vi "子界面-查看某框和报告生成.vi"(2 "测试人":string, 4 "标注图":T1(plugin-control), 5 "部位":string, 6 "产品序号":string, 7 "反射图":T1(plugin-control), 8 "框组":T5(array[cluster]), 9 "框号":dbl format="%#_13g") -> ()   [LabVIEW 2018]
uses:
  <vilib>/addons/database/Connection.llb/DB Tools Open Connec (String).vi
  <vilib>/vision/NI_Vision_Development_Module.lvlib
  <vilib>/addons/database/NI_Database_API.lvlib
panel:
  out "反射图ROI对应区域灰度表":u32[](graph)
  out "?":T1(plugin-control)
  out "Threshold Image":T1(plugin-control)
  out "分层类检测结果":string[][](table)
  out "Threshold Image":T1(plugin-control)
  out "Threshold Image":T1(plugin-control)
  out "反射图ROI的最大灰度值":sgl
  in  "反射法图像-面积阈值设置":T3(array[cluster]) {"Measurement Parameter" items=["Area"]; "下限" min=0 step=1; "上限" min=0 step=1}
  in  "灰度阈值设置":cluster{"下限":dbl, "下限":dbl}(slide)={"下限"=0.0, "下限"=65.10638427734375} scale=0.0..255.0
  in  "保存结果":bool
  in  "Color":u32[](array[colorbox])=[3381759, 16776770, 16777225, 6618880]
  in  "Overlay Type":u16[](array[ring])=[2, 1, 3, 0] items=["Rectangle", "Numbers", "Points", "Lines"]
  in  "Tab Control":T4(tab)
  out "穿透ROI":T1(plugin-control)
  out "Threshold Image":T1(plugin-control)
  out "?":T1(plugin-control)
  out "?":T1(plugin-control)
  out "Threshold Image":T1(plugin-control)
  out "Threshold Image":T1(plugin-control)
  out "弥散测量结果":dbl[][](array[numeric]) format="%.2f"
  in  "分隔符（'\\'代码显示）":string="\t"
  in  "格式字符串":string="%f"
  out "弥散类检测结果":string[][](table)
  out "?":string
  out "面积 (pixels)":i32
  out "写入数据库路径":path
  out "Z值 2":dbl[](array[numeric])
  out "Z值":dbl[](array[numeric])
  out "tables":string[](array[string])
  in  "写入数据库":bool
  out "ROI位置Y":i32
  out "ROI位置X":i32
  out "报告生成路径":path
  in  "格式字符串 2":string="%f"
  in  "分隔符（'\\'代码显示）":string="\t"
  out "分层测量结果":dbl[][](array[numeric]) format="%.2f"
  out "缺陷分类的临界值":sgl format="%#.3f"
  in  "返回 2":bool
  in  "报告生成":bool
  # "所选区域信息"
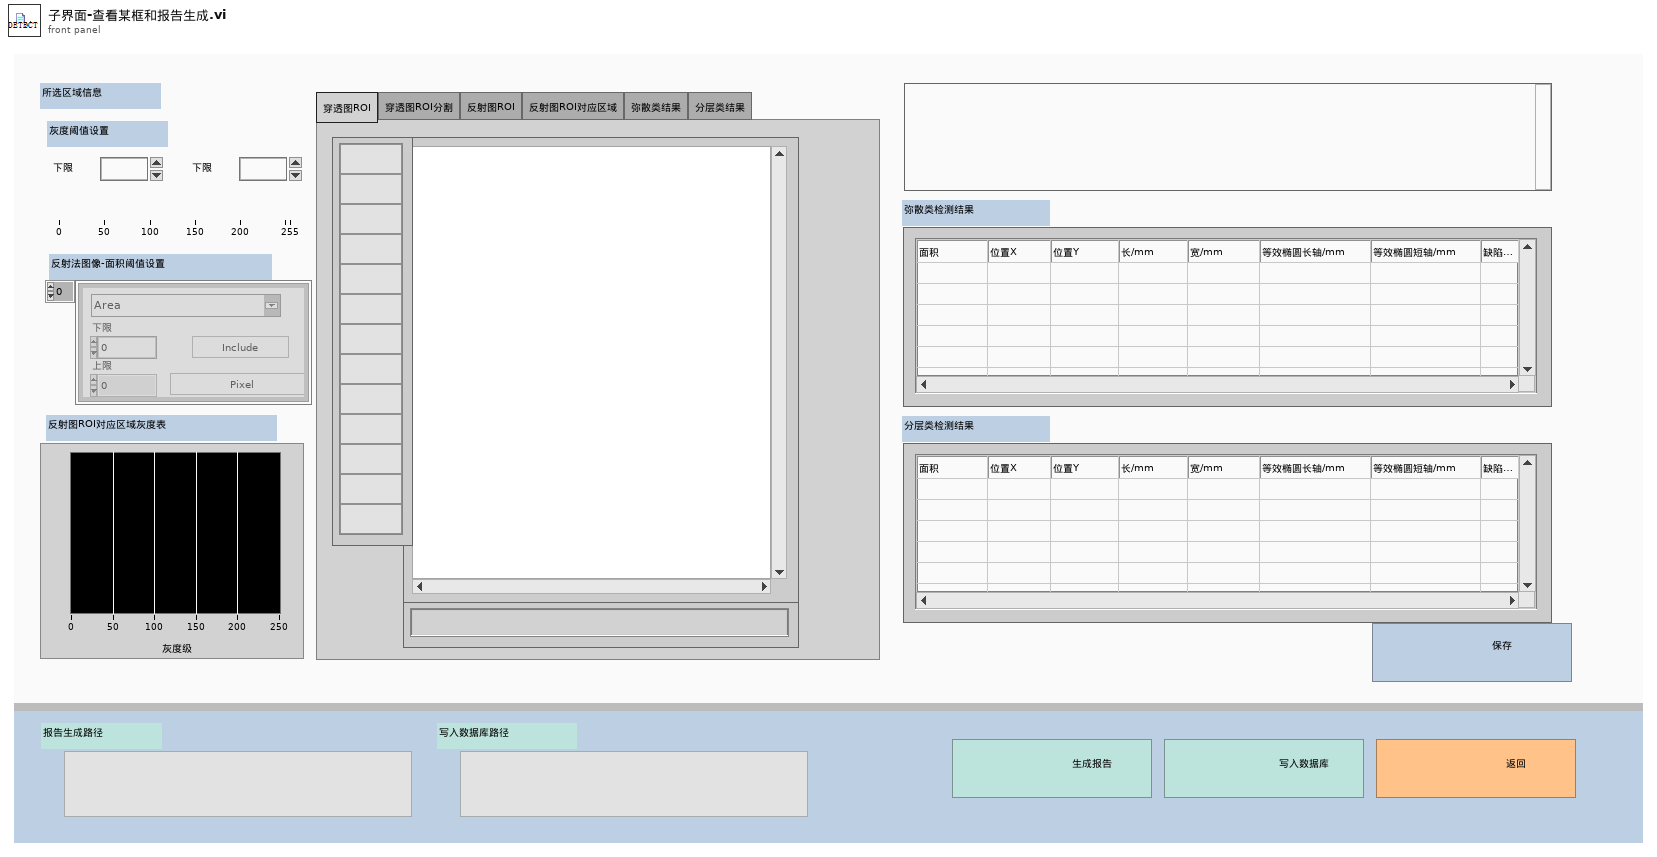
[diagram p1: front panel]
types:
  T1 = typedef "IMAQ Image.ctl" = refnum<image>
  T2 = typedef "Particle Parameters" = i32
  T3 = cluster{"Measurement Parameter":T2, "下限":i32, "上限":i32, "Range":bool, "Measurement Type":bool}[]
  T4 = enum32{"穿透图ROI", "穿透图ROI分割", "反射图ROI", "反射图ROI对应区域", "弥散类结果", "分层类结果"}
  T5 = cluster{"Global Rectangle":i32[], "Contours":cluster{"Contour Type":u32, "ROI Type":u32, "Points":i32[]}[]}[]
  T6 = typedef "Image Type" = u32
  T7 = cluster{"Global Rectangle":i32[], "Contours":cluster{"Contour Type":u32, "ROI Type":u32, "Points":i32[]}[]}
  T8 = cluster{"Pixel Measurements":T2[], "Overlay Type":u16[], "Color":u32[], "反射法图像-面积阈值设置":cluster{"Measurement Parameter":T2, "下限":i32, "上限":i32, "Range":bool, "Measurement Type":bool}[], "灰度阈值设置":cluster{"下限":dbl, "下限":dbl}}
  T9 = cluster{"histogram":u32[], "Minimal Value":sgl, "Maximal Value":sgl, "Starting Value":sgl, "Interval Width":sgl, "Mean Value":sgl, "Standard  Variation":sgl, "Area (pixels)":i32}
  T10 = cluster{"Desired Font (Application)":enum16{"User-specified Font", "Application Font", "System Font", "Dialog Font"}, "[User-specified Font]":cluster{"Font Name":string, "Size":i16, "Strikeout?":bool, "Italic?":bool, "Underline?":bool, "Outline?":bool, "Shadow?":bool, "Bold?":bool, "Rotation Angle":dbl}, "Horizontal Alignment":i16, "Vertical Alignment":i16}
  T11 = typedef "NI_Database_API.lvlib/Conn ObjectReference.ctl" = refnum<k1>
  T12 = cluster{"框号":dbl, "Numeric":dbl, dbl, dbl, "Numeric":dbl, "Numeric":dbl, "Numeric":dbl, "Numeric":dbl, "数值":dbl, string}
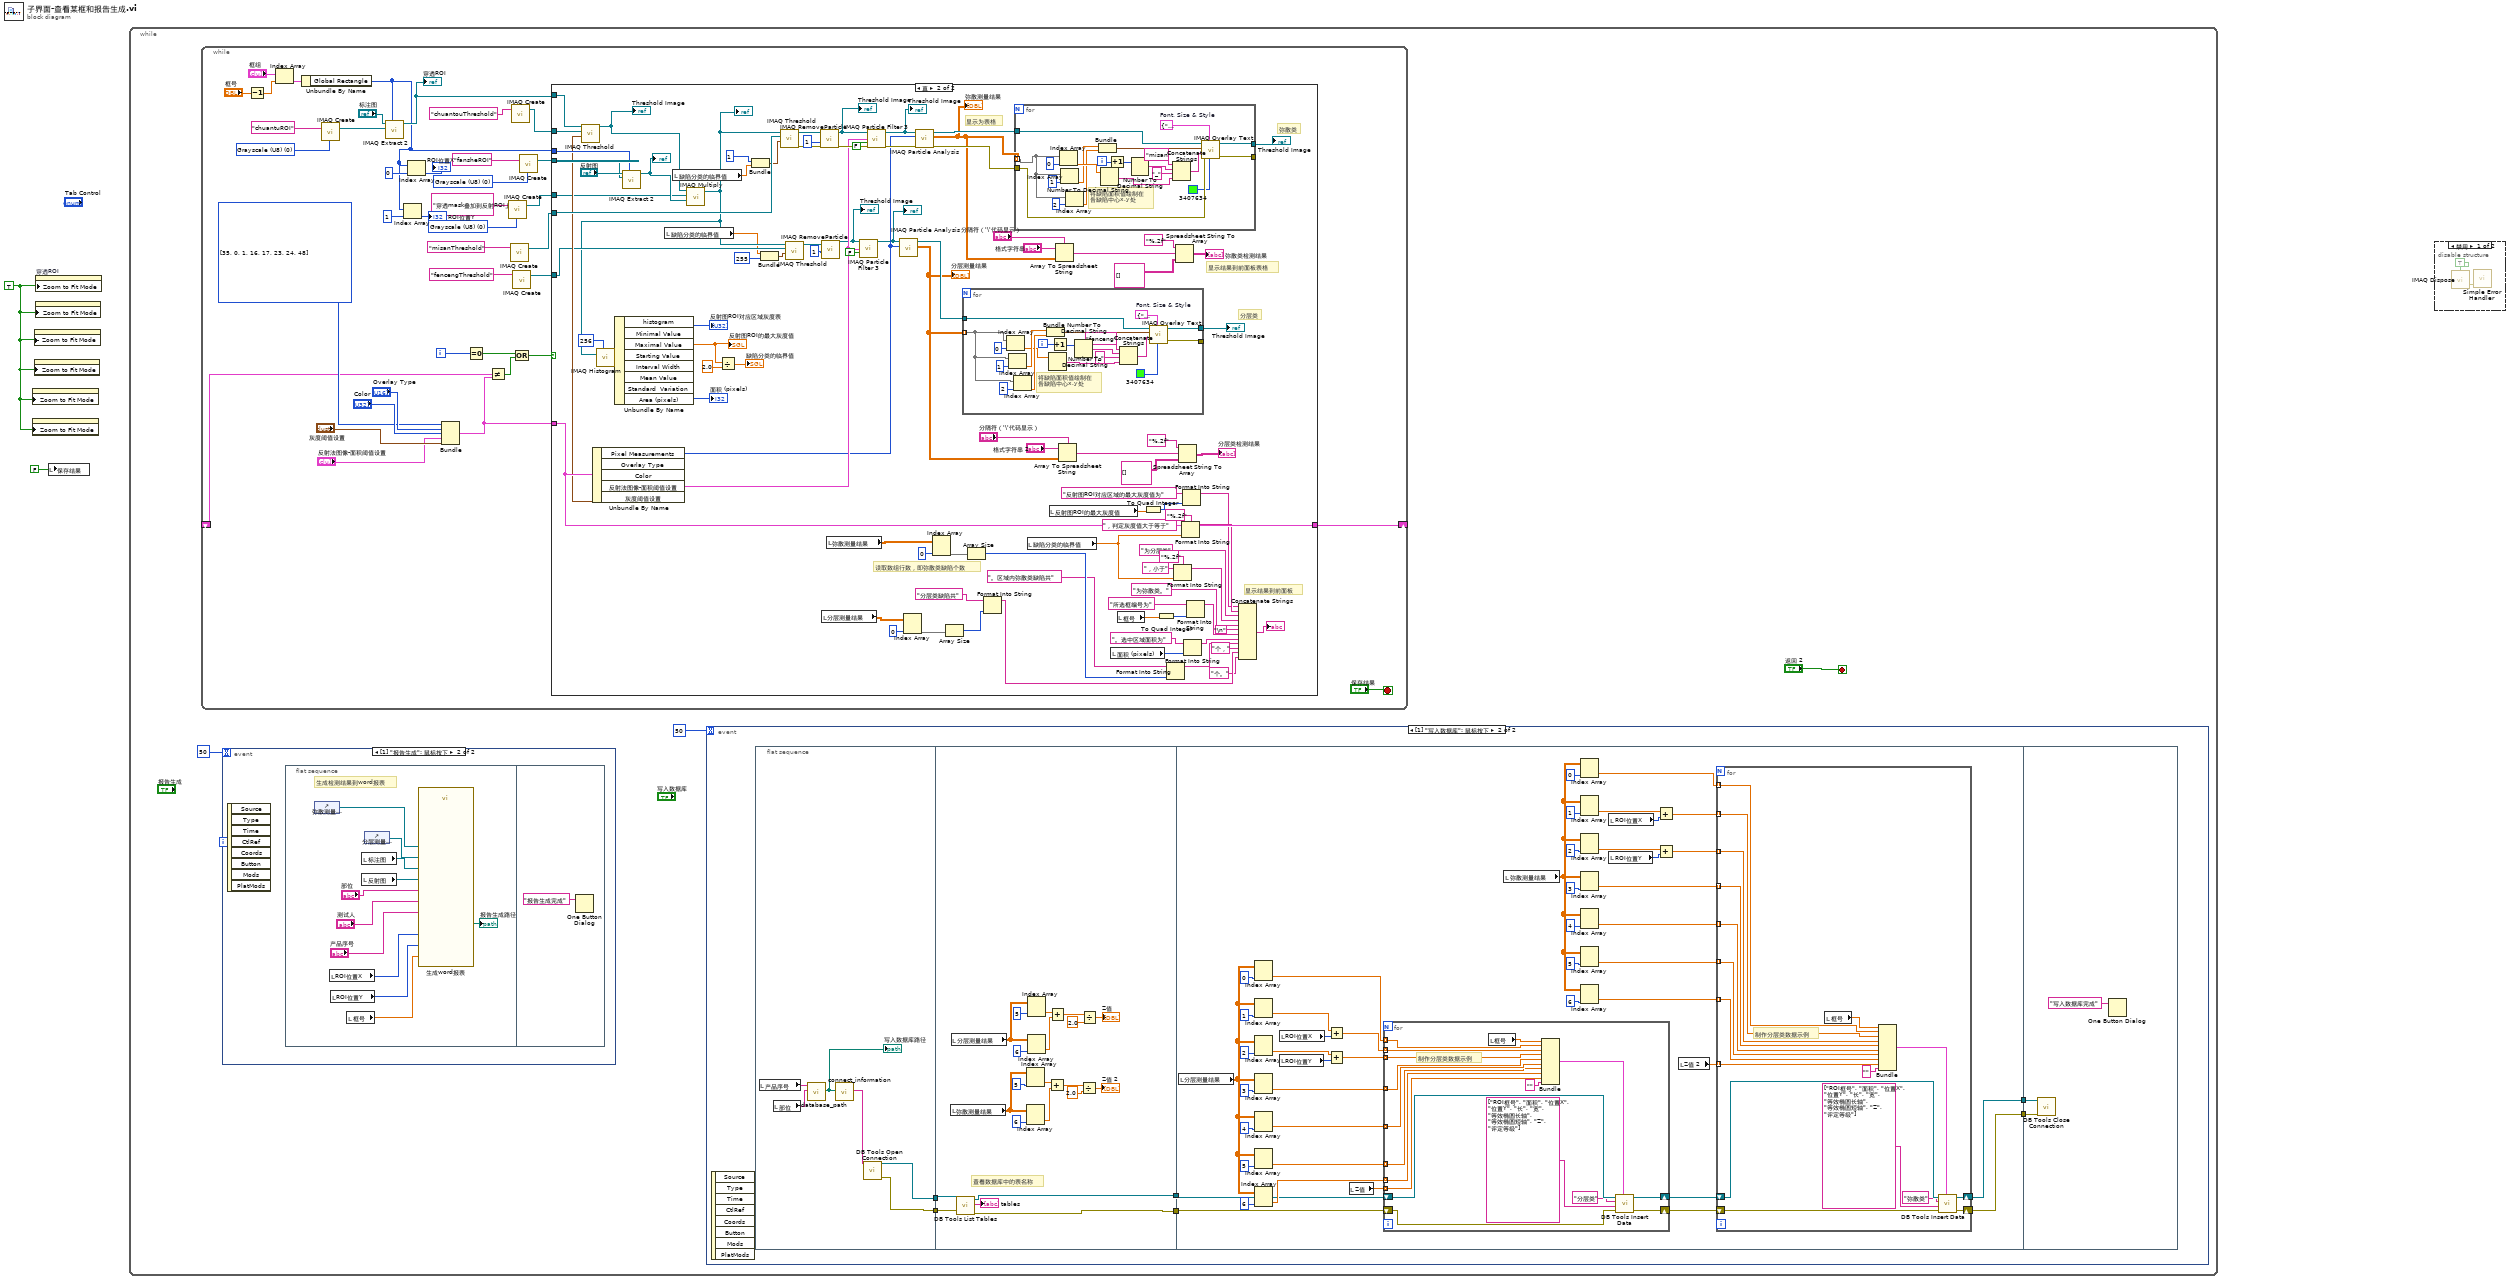
[diagram p0: block diagram]
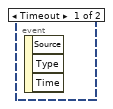
[diagram p3: hidden frame]
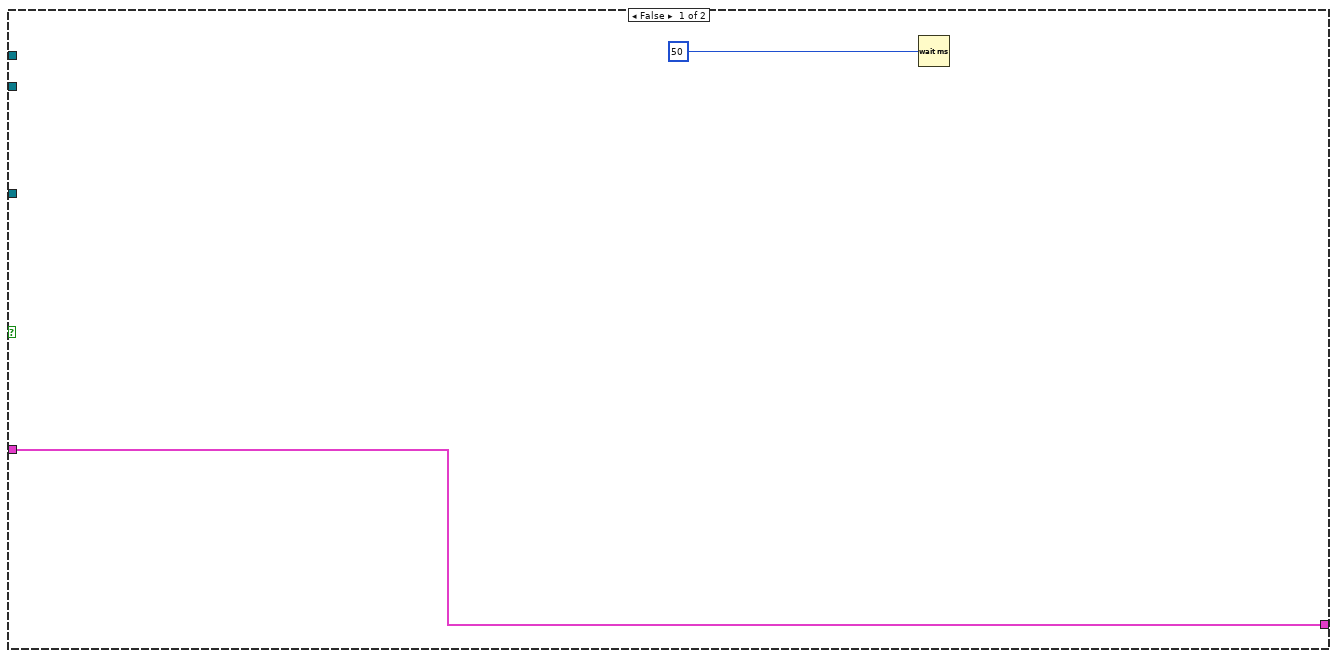
[diagram p4: hidden frame]
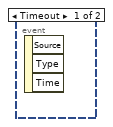
[diagram p5: hidden frame]
diagram:
  w2 = TRUE ("Zoom to Fit Mode")
  n1 = property class="ImageControl"("Zoom to Fit Mode"=w2) -> ()  [unwired: 2 in, 2 out]
  n2 = property class="ImageControl"("Zoom to Fit Mode"=w2) -> ()  [unwired: 2 in, 2 out]
  n3 = property class="ImageControl"("Zoom to Fit Mode"=w2) -> ()  [unwired: 2 in, 2 out]
  n4 = property class="ImageControl"("Zoom to Fit Mode"=w2) -> ()  [unwired: 2 in, 2 out]
  n5 = property class="ImageControl"("Zoom to Fit Mode"=w2) -> ()  [unwired: 2 in, 2 out]
  n6 = property on="穿透ROI" class="ImageControl"("Zoom to Fit Mode"=w2) -> ()  [unwired: 2 in, 2 out]
  n7 = local write "保存结果"(FALSE) -> ()
  n8 = while {
    stop <- "返回 2" stop-if-true
    n9 = while {
      shift-right: [w152] -> _
      shift-left: _ -> [w151]
      i -> [w156]
      stop <- "保存结果" stop-if-true
      w131 = T6 0 items=["Grayscale (U8)", "Grayscale (I16)", "Grayscale (SGL)", "Complex (CSG)", "RGB (U32)", "HSL (U32)", "RGB (U64)", "Grayscale (U16)"] ("Image Type")
      w137 = T6 0 items=["Grayscale (U8)", "Grayscale (I16)", "Grayscale (SGL)", "Complex (CSG)", "RGB (U32)", "HSL (U32)", "RGB (U64)", "Grayscale (U16)"] ("Image Type")
      w143 = T6 0 items=["Grayscale (U8)", "Grayscale (I16)", "Grayscale (SGL)", "Complex (CSG)", "RGB (U32)", "HSL (U32)", "RGB (U64)", "Grayscale (U16)"] ("Image Type")
      w158 = T2[] [35, 0, 1, 16, 17, 23, 24, 48] items=["Center of Mass X", "Center of Mass Y", "First Pixel X", "First Pixel Y", "Bounding Rect Left", "Bounding Rect Top", "Bounding Rect Right", "Bounding Rect Bottom", "Max Feret Diameter Start X", "Max Feret Diameter Start Y", "Max Feret Diameter End X", "Max Feret Diameter End Y", "Max Horiz. Segment Length Left", "Max Horiz. Segment Length Right", "Max Horiz. Segment Length Row", "-", "Bounding Rect Width", "Bounding Rect Height", "Bounding Rect Diagonal", "Perimeter", "Convex Hull Perimeter", "Holes' Perimeter", "Max Feret Diameter", "Equivalent Ellipse Major Axis", "Equivalent Ellipse Minor Axis", "Equivalent Ellipse Minor Axis (Feret)", "Equivalent Rect Long Side", "Equivalent Rect Short Side", "Equivalent Rect Diagonal", "Equivalent Rect Short Side (Feret)", "Average Horiz. Segment Length", "Average Vert. Segment Length", "Hydraulic Radius", "Waddel Disk Diameter", "-", "Area", "Holes' Area", "Particle & Holes' Area", "Convex Hull Area", "Image Area", "-", "Number of Holes", "Number of Horiz. Segments", "Number of Vert. Segments", "-", "Orientation", "Max Feret Diameter Orientation", "-", "% Area/Image Area", "% Area/(Particle & Holes' Area)", "Ratio of Equivalent Ellipse Axes", "Ratio of Equivalent Rect Sides", "-", "Elongation Factor", "Compactness Factor", "Heywood Circularity Factor", "Type Factor", "-", "Sum X", "Sum Y", "Sum XX", "Sum XY", "Sum YY", "Sum XXX", "Sum XXY", "Sum XYY", "Sum YYY", "-", "Moment of Inertia XX", "Moment of Inertia XY", "Moment of Inertia YY", "Moment of Inertia XXX", "Moment of Inertia XXY", "Moment of Inertia XYY", "Moment of Inertia YYY", "Norm. Moment of Inertia XX", "Norm. Moment of Inertia XY", "Norm. Moment of Inertia YY", "Norm. Moment of Inertia XXX", "Norm. Moment of Inertia XXY", "Norm. Moment of Inertia XYY", "Norm. Moment of Inertia YYY", "Hu Moment 1", "Hu Moment 2", "Hu Moment 3", "Hu Moment 4", "Hu Moment 5", "Hu Moment 6", "Hu Moment 7"] ("Pixel Measurements")
      n10 = Decrement(x="框号") -> (x-1=w145:dbl)
      n11 = Index Array(array="框组", index=w145) -> (element=w147:T7)
      n12 = Unbundle By Name(w147) -> ("Global Rectangle"=w123:i32[])
      n13 = call "IMAQ Create"("Image Name"="chuantuROI", "Image Type"=w143) -> ("New Image"=w146:T1)  [unwired: 3 in, 1 out]
      n14 = call "IMAQ Extract 2"("Optional Rectangle"=w123, "Image Dst"=w146, "Image Src"="标注图") -> ("Image Dst Out"=w134:T1)  [unwired: 7 in, 1 out]
      "穿透ROI" <- w134
      n15 = Index Array(array=w123, index=1 ("索引")) -> (element=→"ROI位置Y":i32)
      n16 = Index Array(array=w123, index=0 ("索引")) -> (element=→"ROI位置X":i32)
      n17 = Bundle("Pixel Measurements"=w158, "Overlay Type"="Overlay Type", "Color"="Color", "反射法图像-面积阈值设置"="反射法图像-面积阈值设置", "灰度阈值设置"="灰度阈值设置") -> (w135:T8)  [unwired: 1 in]
      n18 = Equal To 0?(x=w156) -> (x = 0?=w155:bool)
      n19 = Not Equal?(x=w151, y=w135) -> (x != y?=w154:bool)
      n20 = call "IMAQ Create"("Image Name"="穿透mask叠加到反射ROI上", "Image Type"=w131) -> ("New Image"=w130:T1)  [unwired: 3 in, 1 out]
      n21 = call "IMAQ Create"("Image Name"="misanThreshold") -> ("New Image"=w129:T1)  [unwired: 4 in, 1 out]
      n22 = call "IMAQ Create"("Image Name"="chuantouThreshold") -> ("New Image"=w139:T1)  [unwired: 4 in, 1 out]
      n23 = call "IMAQ Create"("Image Name"="fencengThreshold") -> ("New Image"=w127:T1)  [unwired: 4 in, 1 out]
      n24 = Compound Arithmetic op=OR(w155, w154) -> (w153:bool)
      n25 = call "IMAQ Create"("Image Name"="fansheROI", "Image Type"=w137) -> ("New Image"=w136:T1)  [unwired: 3 in, 1 out]
      n26 = case shown="真" w153 {
        tunnel: w135 -> [w161 w224]
        tunnel: [w161 w224] -> w152
        tunnel: w139 -> [_ w232]
        tunnel: w134 -> [_ w222]
        tunnel: w136 -> [_ w230]
        tunnel: w123 -> [_ w229]
        tunnel: w129 -> [_ w228]
        tunnel: w130 -> [_ w219]
        tunnel: w127 -> [_ w194]
        frame False {
          n27 = Wait (ms)(milliseconds to wait=u32 50) -> ()  [unwired: 1 out]
        }
        frame True {
          # "分层类"
          # "弥散类"
          # "显示结果到前面板"
          # "读取数组行数，即弥散类缺陷个数"
          # "显示结果到前面板表格"
          # "显示为表格"
          n28 = Unbundle By Name(w224) -> ("Pixel Measurements"=w185:T2[], "反射法图像-面积阈值设置"=w187:T3, "灰度阈值设置"=w223:cluster{"下限":dbl, "下限":dbl})  [unwired: 2 out]
          n29 = call "IMAQ Threshold"("Range"=w223, "Image Dst"=w232, "Image Src"=w222) -> ("Image Dst Out"=w221:T1)  [unwired: 3 in, 5 out]
          "Threshold Image" <- w221
          n30 = call "IMAQ Extract 2"("Optional Rectangle"=w229, "Image Dst"=w230, "Image Src"="反射图") -> ("Image Dst Out"=w220:T1)  [unwired: 7 in, 1 out]
          "?" <- w220
          n31 = local read "缺陷分类的临界值"() -> (w190:sgl)
          n32 = local read "缺陷分类的临界值"() -> (w201:sgl)
          n33 = call "IMAQ Multiply"("Image Src A"=w221, "Image Dst"=w219, "Image Src B"=w220) -> ("Image Dst Out"=w193:T1)  [unwired: 4 in, 1 out]
          "?" <- w193
          n34 = call "IMAQ Histogram"("Number of Classes"=256, "Image"=w193) -> ("Histogram Report"=w227:T9)  [unwired: 8 in, 1 out]
          n35 = Unbundle By Name(w227) -> ("histogram"=→"反射图ROI对应区域灰度表":u32[], "Maximal Value"=w215:sgl, "Area (pixels)"=→"面积 (pixels)":i32)  [unwired: 5 out]
          "反射图ROI的最大灰度值" <- w215
          n36 = Divide(x=w215, y=sgl 2.0) -> (x/y=→"缺陷分类的临界值":sgl)
          n37 = Bundle(1, "缺陷分类的临界值"=w201) -> (w200:cluster{i32, "缺陷分类的临界值":sgl})  [unwired: 1 in]
          n38 = Bundle("缺陷分类的临界值"=w190, 255) -> (w192:cluster{"缺陷分类的临界值":sgl, i32})  [unwired: 1 in]
          n39 = call "IMAQ Threshold"("Range"=w200, "Image Dst"=w228, "Image Src"=w193) -> ("error out"=w256:errorcluster, "Image Dst Out"=w233:T1)  [unwired: 3 in, 4 out]
          n40 = call "IMAQ Threshold"("Range"=w192, "Image Dst"=w194, "Image Src"=w193) -> ("Image Dst Out"=w189:T1)  [unwired: 3 in, 5 out]
          n41 = call "IMAQ RemoveParticle"("error in (no error)"=w256, "Number of Erosion"=1, "Image Src"=w233) -> ("error out"=w255:errorcluster, "Image Dst Out"=w198:T1)  [unwired: 7 in]
          "Threshold Image" <- w198
          n42 = local read "分层测量结果"() -> (w173:dbl[][])
          n43 = call "IMAQ RemoveParticle"("Number of Erosion"=1, "Image Src"=w189) -> ("Image Dst Out"=w168:T1)  [unwired: 8 in, 1 out]
          "Threshold Image" <- w168
          n44 = local read "弥散测量结果"() -> (w195:dbl[][])
          n45 = call "IMAQ Particle Filter 3"("Image Src"=w168, "Selection Values"=w187, "Keep/Remove Particles (F)"=FALSE) -> ("Image Dst Out"=w167:T1)  [unwired: 10 in, 2 out]
          "?" <- w167
          n46 = call "IMAQ Particle Filter 3"("Image Src"=w198, "Selection Values"=w187, "Keep/Remove Particles (F)"=FALSE, "error in (no error)"=w255) -> ("Image Dst Out"=w197:T1, "error out"=w254:errorcluster)  [unwired: 9 in, 1 out]
          "Threshold Image" <- w197
          n47 = call "IMAQ Particle Analysis"("Pixel Measurements"=w185, "Image"=w167) -> ("Particle Measurements (Pixels)"=w179:dbl[][], "Image Out (duplicate)"=w184:T1)  [unwired: 4 in, 4 out]
          "分层测量结果" <- w179
          n48 = Index Array(array=w173, index (col)=0 ("禁用的索引 (列)")) -> (element=w175:dbl[])  [unwired: 1 in]
          n49 = call "IMAQ Particle Analysis"("error in (no error)"=w254, "Pixel Measurements"=w185, "Image"=w197) -> ("error out"=w252:errorcluster, "Particle Measurements (Pixels)"=w234:dbl[][], "Image Out (duplicate)"=w253:T1)  [unwired: 3 in, 3 out]
          "弥散测量结果" <- w234
          n50 = Index Array(array=w195, index (col)=0 ("禁用的索引 (列)")) -> (element=w240:dbl[])  [unwired: 1 in]
          n51 = Array Size(array=w175) -> (size(s)=w171:i32)
          n52 = for {
            tunnel: [w278] -> _
            tunnel: [w277] -> w183
            tunnel: w184 -> [w264]
            tunnel: w179 -> [w262] mode=indexing
            i -> [w259]
            w275 = T10 {"Desired Font (Application)"=enum."Application Font", "[User-specified Font]"={"Font Name"="", "Size"=12, "Strikeout?"=FALSE, "Italic?"=FALSE, "Underline?"=FALSE, "Outline?"=FALSE, "Shadow?"=FALSE, "Bold?"=FALSE, "Rotation Angle"=0.0}, "Horizontal Alignment"=0, "Vertical Alignment"=0}  # Font, Size & Style
            # "将缺陷面积值绘制在\n各缺陷中心x,y处"
            n53 = Index Array(array=w262, index=0 ("索引")) -> (element=w261:dbl)
            n54 = Index Array(array=w262, index=1 ("索引")) -> (element=w272:dbl)
            n55 = Index Array(array=w262, index=2 ("索引")) -> (element=w270:dbl)
            n56 = Bundle("Numeric"=w272, "Numeric"=w270) -> (w263:cluster{"Numeric":dbl, "Numeric":dbl})  [unwired: 1 in]
            n57 = Number To Decimal String(number=w261) -> (decimal integer string=w267:string)  [unwired: 1 in]
            n58 = Increment(x=w259) -> (x+1=w260:i32)
            n59 = Number To Decimal String(number=w260) -> (decimal integer string=w269:string)  [unwired: 1 in]
            n60 = Concatenate Strings("fenceng" ("字符串"), w269, "_", w267) -> (w266:string)
            n61 = call "IMAQ Overlay Text"("Text Color (black)"=u32 3407634, "Font, Size & Style"=w275, "String"=w266, "Origin"=w263, "Image"=w264) -> ("error out"=w278:errorcluster, "Image Out"=w277:T1)  [unwired: 5 in]
          }
          "Threshold Image" <- w183
          n62 = Array Size(array=w240) -> (size(s)=w242:i32)
          n63 = Format Into String(initial string="分层类缺陷共" ("初始字符串"), w171) -> (resulting string=w170:string)  [unwired: 2 in, 1 out]
          n64 = for {
            tunnel: w252 -> [w299]
            tunnel: [w298] -> _
            tunnel: [w297] -> w199
            tunnel: w253 -> [w295]
            tunnel: w234 -> [w288] mode=indexing
            i -> [w280]
            w294 = T10 {"Desired Font (Application)"=enum."Application Font", "[User-specified Font]"={"Font Name"="", "Size"=12, "Strikeout?"=FALSE, "Italic?"=FALSE, "Underline?"=FALSE, "Outline?"=FALSE, "Shadow?"=FALSE, "Bold?"=FALSE, "Rotation Angle"=0.0}, "Horizontal Alignment"=0, "Vertical Alignment"=0}  # Font, Size & Style
            # "将缺陷面积值绘制在\n各缺陷中心x,y处"
            n65 = Index Array(array=w288, index=0 ("索引")) -> (element=w293:dbl)
            n66 = Index Array(array=w288, index=1 ("索引")) -> (element=w290:dbl)
            n67 = Index Array(array=w288, index=2 ("索引")) -> (element=w287:dbl)
            n68 = Bundle("Numeric"=w290, "Numeric"=w287) -> (w286:cluster{"Numeric":dbl, "Numeric":dbl})  [unwired: 1 in]
            n69 = Number To Decimal String(number=w293) -> (decimal integer string=w283:string)  [unwired: 1 in]
            n70 = Increment(x=w280) -> (x+1=w279:i32)
            n71 = Number To Decimal String(number=w279) -> (decimal integer string=w285:string)  [unwired: 1 in]
            n72 = Concatenate Strings("misan" ("字符串"), w285, "_", w283) -> (w282:string)
            n73 = call "IMAQ Overlay Text"("Text Color (black)"=u32 3407634, "Font, Size & Style"=w294, "error in (no error)"=w299, "String"=w282, "Origin"=w286, "Image"=w295) -> ("error out"=w298:errorcluster, "Image Out"=w297:T1)  [unwired: 4 in]
          }
          "Threshold Image" <- w199
          n74 = local read "缺陷分类的临界值"() -> (w165:sgl)
          n75 = local read "反射图ROI的最大灰度值"() -> (w218:sgl)
          n76 = Array To Spreadsheet String(delimiter (Tab)="分隔符（'\\'代码显示）", array=w234, 3:"格式字符串") -> (spreadsheet string=w248:string)
          n77 = Array To Spreadsheet String(delimiter (Tab)="分隔符（'\\'代码显示）", array=w179, 3:"格式字符串 2") -> (spreadsheet string=w178:string)
          n78 = local read "面积 (pixels)"() -> (w239:i32)
          n79 = local read "框号"() -> (w244:dbl)
          n80 = To Quad Integer(1:w218) -> (0:w217:i64)
          n81 = To Quad Integer(1:w244) -> (0:w243:i64)
          n82 = Format Into String(initial string="。区域内弥散类缺陷共" ("初始字符串"), w242) -> (resulting string=w204:string)  [unwired: 2 in, 1 out]
          n83 = Format Into String(format string="%.2f" ("格式字符串"), initial string="，小于" ("初始字符串"), w165) -> (resulting string=w209:string)  [unwired: 1 in, 1 out]
          n84 = Spreadsheet String To Array(format string="%.2f", spreadsheet string=w248, array type (2D Dbl)=string[][] [] ("Array")) -> (array=→"弥散类检测结果":string[][])  [unwired: 1 in]
          n85 = Spreadsheet String To Array(format string="%.2f", spreadsheet string=w178, array type (2D Dbl)=string[][] [] ("Array")) -> (array=→"分层类检测结果":string[][])  [unwired: 1 in]
          n86 = Format Into String(format string="%.2f" ("格式字符串"), initial string="，判定灰度值大于等于" ("初始字符串"), w165) -> (resulting string=w207:string)  [unwired: 1 in, 1 out]
          n87 = Format Into String(initial string="反射图ROI对应区域的最大灰度值为" ("初始字符串"), w217) -> (resulting string=w206:string)  [unwired: 2 in, 1 out]
          n88 = Format Into String(initial string="。选中区域面积为" ("字符串"), w239) -> (resulting string=w205:string)  [unwired: 2 in, 1 out]
          n89 = Format Into String(initial string="所选框编号为" ("初始字符串"), w243) -> (resulting string=w245:string)  [unwired: 2 in, 1 out]
          n90 = Concatenate Strings(w206, w207, "为分层类" ("初始字符串"), w209, "为弥散类。" ("初始字符串"), "\n", w245, w205, w204, "个，" ("字符串"), w170, "个。" ("字符串")) -> (→"?":string)
        }
      }
    }
    n91 = event shown="[1] \"报告生成\": 鼠标按下" {
      selector: _ -> [_ _]
      dyn-events: _ -> [_ _]
      timeout: 50 -> [_ _]
      event Timeout {
        n92 = event-data() -> ()  [unwired: 1 in, 3 out]
      }
      event "报告生成": Mouse Down {
        n93 = event-data() -> ()  [unwired: 1 in, 8 out]
        n94 = flat-sequence {
          frame #0 {
            # "生成检测结果到word报表"
            n95 = control-ref of="弥散测量结果"() -> (w308:refnum<vi>)
            n96 = local read "ROI位置X"() -> (w305:i32)
            n97 = local read "ROI位置Y"() -> (w304:i32)
            n98 = local read "框号"() -> (w303:dbl)
            n99 = local read "标注图"() -> (w309:T1)
            n100 = local read "反射图"() -> (w310:T1)
            n101 = control-ref of="分层测量结果"() -> (w307:refnum<vi>)
            n102 = call "生成word报表.vi"("Array输入"=w308, "产品序号"="产品序号", "标注图"=w310, "Array输入 2"=w307, "测试人"="测试人", "部位"="部位", "ROI左上角X"=w305, "ROI左上角Y"=w304, "反射图"=w309, "框号"=w303) -> ("报告生成路径"=→"报告生成路径":path)  [unwired: 9 in]
          }
          frame #1 {
            n103 = One Button Dialog(message="报告生成完成" ("消息")) -> ()  [unwired: 1 in, 1 out]
          }
        }
      }
    }
    n104 = event shown="[1] \"写入数据库\": 鼠标按下" {
      selector: _ -> [_ _]
      dyn-events: _ -> [_ _]
      timeout: 50 -> [_ _]
      event Timeout {
        n105 = event-data() -> ()  [unwired: 1 in, 3 out]
      }
      event "写入数据库": Mouse Down {
        n106 = event-data() -> ()  [unwired: 1 in, 8 out]
        n107 = flat-sequence {
          tunnel: [w16] -> w11
          tunnel: [w15] -> w10
          tunnel: w11 -> [w19]
          tunnel: [w36] -> w9
          tunnel: w10 -> [w37]
          tunnel: [w18] -> w6
          tunnel: w9 -> [w84]
          tunnel: [w54] -> w8
          tunnel: [w53] -> w7
          tunnel: w6 -> [w39]
          tunnel: w8 -> [w121]
          tunnel: w7 -> [w120]
          frame #0 {
            n108 = local read "产品序号"() -> (w14:string)
            n109 = local read "部位"() -> (w13:string)
            n110 = call "database_path.vi"("部位"=w13, "产品序号"=w14) -> ("database path"=w12:path)  [unwired: 9 in]
            "写入数据库路径" <- w12
            n111 = call "connect_information.vi"("路径"=w12) -> ("connect info"=w17:string)  [unwired: 10 in]
            n112 = call-poly <vilib>:"DB Tools Open Connection.vi"("connection information"=w17) -> ("error out"=w15:errorcluster, "connection reference"=w16:T11)  [unwired: 7 in]
          }
          frame #1 {
            # "查看数据库中的表名称"
            n113 = local read "弥散测量结果"() -> (w20:dbl[][])
            n114 = local read "分层测量结果"() -> (w32:dbl[][])
            n115 = call <vilib>:"DB Tools List Tables.vi"("error in (no error)"=w37, "connection reference"=w19) -> ("error out"=w36:errorcluster, "tables"=→"tables":string[], "connection reference out"=w18:T11)  [unwired: 3 in]
            n116 = Index Array(array=w20, index (col)=5 ("禁用的索引 (列)")) -> (element=w24:dbl[])  [unwired: 1 in]
            n117 = Index Array(array=w20, index (col)=6 ("索引 (列)")) -> (element=w23:dbl[])  [unwired: 1 in]
            n118 = Index Array(array=w32, index (col)=5 ("禁用的索引 (列)")) -> (element=w31:dbl[])  [unwired: 1 in]
            n119 = Index Array(array=w32, index (col)=6 ("索引 (列)")) -> (element=w30:dbl[])  [unwired: 1 in]
            n120 = Add(x=w24, y=w23) -> (x+y=w22:dbl[])
            n121 = Add(x=w31, y=w30) -> (x+y=w29:dbl[])
            n122 = Divide(x=w22, y=2.0) -> (x/y=→"Z值 2":dbl[])
            n123 = Divide(x=w29, y=2.0) -> (x/y=→"Z值":dbl[])
          }
          frame #2 {
            n124 = local read "分层测量结果"() -> (w75:dbl[][])
            n125 = Index Array(array=w75, index (col)=0 ("禁用的索引 (列)")) -> (element=w76:dbl[])  [unwired: 1 in]
            n126 = Index Array(array=w75, index (col)=1 ("禁用的索引 (列)")) -> (element=w66:dbl[])  [unwired: 1 in]
            n127 = Index Array(array=w75, index (col)=2 ("禁用的索引 (列)")) -> (element=w69:dbl[])  [unwired: 1 in]
            n128 = Index Array(array=w75, index (col)=3 ("禁用的索引 (列)")) -> (element=w74:dbl[])  [unwired: 1 in]
            n129 = Index Array(array=w75, index (col)=4 ("禁用的索引 (列)")) -> (element=w72:dbl[])  [unwired: 1 in]
            n130 = Index Array(array=w75, index (col)=5 ("禁用的索引 (列)")) -> (element=w71:dbl[])  [unwired: 1 in]
            n131 = Index Array(array=w75, index (col)=6 ("禁用的索引 (列)")) -> (element=w73:dbl[])  [unwired: 1 in]
            n132 = local read "ROI位置X"() -> (w65:i32)
            n133 = local read "ROI位置Y"() -> (w68:i32)
            n134 = Add(x=w66, y=w65) -> (x+y=w64:dbl[])
            n135 = Add(x=w69, y=w68) -> (x+y=w67:dbl[])
            n136 = local read "Z值"() -> (w70:dbl[])
            n137 = for {
              shift-right: [w117] -> w41
              shift-left: w39 -> [w118]
              shift-right: [w115] -> w40
              shift-left: w84 -> [w116]
              tunnel: w76 -> [w110] mode=indexing
              tunnel: w74 -> [w109] mode=indexing
              tunnel: w72 -> [w107] mode=indexing
              tunnel: w71 -> [w106] mode=indexing
              tunnel: w73 -> [w108] mode=indexing
              tunnel: w70 -> [w105] mode=indexing
              tunnel: w67 -> [w104] mode=indexing
              tunnel: w64 -> [w103] mode=indexing
              # "制作分层类数据示例"
              n138 = local read "框号"() -> (w102:dbl)
              n139 = Bundle("框号"=w102, "Numeric"=w110, w103, w104, "Numeric"=w109, "Numeric"=w107, "Numeric"=w106, "Numeric"=w108, "数值"=w105, "") -> (w111:T12)  [unwired: 1 in]
              n140 = call <vilib>:"DB Tools Insert Data.vi"("data"=w111, "error in (no error)"=w116, "columns"=string[] ["ROI框号", "面积", "位置X", "位置Y", "长", "宽", "等效椭圆长轴", "等效椭圆短轴", "Z", "评定等级"], "table"="分层类", "connection reference"=w118) -> ("error out"=w115:errorcluster, "connection reference out"=w117:T11)  [unwired: 5 in]
            }
            n141 = local read "弥散测量结果"() -> (w55:dbl[][])
            n142 = Index Array(array=w55, index (col)=0 ("禁用的索引 (列)")) -> (element=w56:dbl[])  [unwired: 1 in]
            n143 = Index Array(array=w55, index (col)=1 ("禁用的索引 (列)")) -> (element=w52:dbl[])  [unwired: 1 in]
            n144 = Index Array(array=w55, index (col)=2 ("禁用的索引 (列)")) -> (element=w48:dbl[])  [unwired: 1 in]
            n145 = Index Array(array=w55, index (col)=3 ("禁用的索引 (列)")) -> (element=w46:dbl[])  [unwired: 1 in]
            n146 = Index Array(array=w55, index (col)=4 ("禁用的索引 (列)")) -> (element=w45:dbl[])  [unwired: 1 in]
            n147 = Index Array(array=w55, index (col)=5 ("禁用的索引 (列)")) -> (element=w44:dbl[])  [unwired: 1 in]
            n148 = Index Array(array=w55, index (col)=6 ("禁用的索引 (列)")) -> (element=w43:dbl[])  [unwired: 1 in]
            n149 = local read "ROI位置X"() -> (w51:i32)
            n150 = local read "ROI位置Y"() -> (w49:i32)
            n151 = Add(x=w52, y=w51) -> (x+y=w50:dbl[])
            n152 = Add(x=w48, y=w49) -> (x+y=w47:dbl[])
            n153 = local read "Z值 2"() -> (w42:dbl[])
            n154 = for {
              shift-right: [w100] -> w54
              shift-left: w41 -> [w101]
              shift-right: [w98] -> w53
              shift-left: w40 -> [w99]
              tunnel: w56 -> [w93] mode=indexing
              tunnel: w46 -> [w92] mode=indexing
              tunnel: w47 -> [w91] mode=indexing
              tunnel: w50 -> [w90] mode=indexing
              tunnel: w45 -> [w88] mode=indexing
              tunnel: w44 -> [w87] mode=indexing
              tunnel: w43 -> [w86] mode=indexing
              tunnel: w42 -> [w85] mode=indexing
              # "制作分层类数据示例"
              n155 = local read "框号"() -> (w89:dbl)
              n156 = Bundle("框号"=w89, "Numeric"=w93, w90, w91, "Numeric"=w92, "Numeric"=w88, "Numeric"=w87, "Numeric"=w86, "数值"=w85, "") -> (w94:T12)  [unwired: 1 in]
              n157 = call <vilib>:"DB Tools Insert Data.vi"("data"=w94, "error in (no error)"=w99, "columns"=string[] ["ROI框号", "面积", "位置X", "位置Y", "长", "宽", "等效椭圆长轴", "等效椭圆短轴", "Z", "评定等级"], "table"="弥散类", "connection reference"=w101) -> ("error out"=w98:errorcluster, "connection reference out"=w100:T11)  [unwired: 5 in]
            }
          }
          frame #3 {
            n158 = call <vilib>:"DB Tools Close Connection.vi"("error in (no error)"=w120, "connection reference"=w121) -> ()  [unwired: 5 in, 1 out]
            n159 = One Button Dialog(message="写入数据库完成" ("消息")) -> ()  [unwired: 1 in, 1 out]
          }
        }
      }
    }
  }
  n160 = disable-structure shown="禁用" {
    frame Disabled {
      n161 = call "IMAQ Dispose"("All Images? (No)"=TRUE) -> ("error out"=w313:errorcluster)  [unwired: 5 in]
      n162 = call <vilib>:"Simple Error Handler.vi"("error in (no error)"=w313) -> ()  [unwired: 4 in, 5 out]
    }
    frame Enabled {
    }
  }
